vi "Clean Buffers.vi"(8 "error in (no error)":errorcluster, 11 "State In":T1) -> (0 "error out":errorcluster, 3 "State Out":T1)   [LabVIEW 2020, in "TDMS DAQ.lvlib" / "TDMS DAQ.lvclass"]
uses:
  TDMS DAQ.lvclass
  Helper Loop State.ctl
  <vilib>/Natan Biesmans/G2CPU GPU and CPU HPC Toolkit/G2CPU Libraries/Async IO/DMA Manager/DMA Manager.lvclass
  Configure TDMS DAQ.ctl
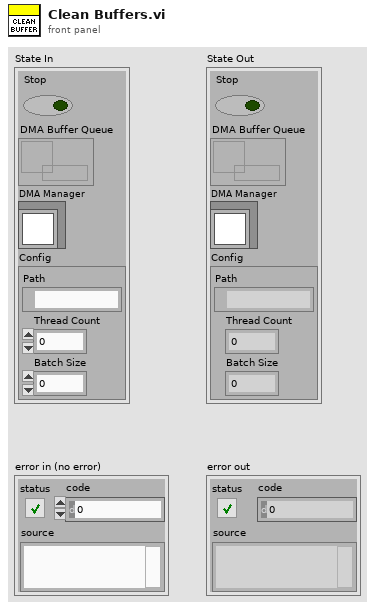
[diagram p1: front panel]
types:
  T1 = typedef "TDMS DAQ.lvlib/TDMS DAQ.lvclass/Helper Loop State.ctl" = cluster{"Stop":bool, "DMA Buffer Queue":refnum<queue>, "DMA Manager":refnum<class "DMA Manager.lvclass">, "Config":T2}
  T2 = typedef "TDMS DAQ.lvlib/TDMS DAQ.lvclass/Configure TDMS DAQ.ctl" = cluster{"Path":path, "Thread Count":i32, "Batch Size":i32}
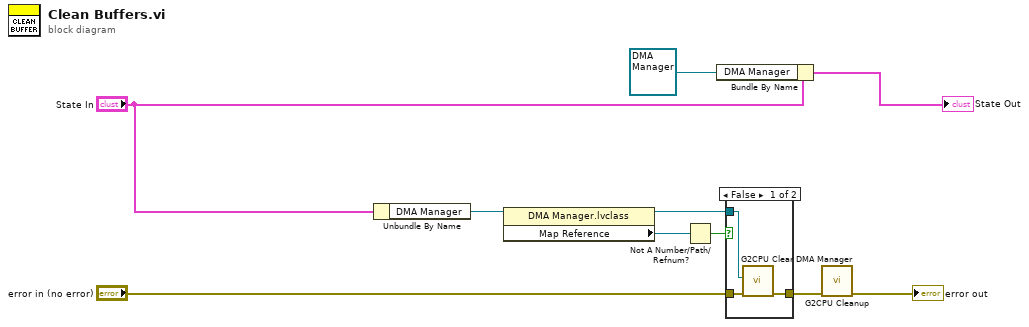
[diagram p0: block diagram]
diagram:
  n1 = Unbundle By Name("State In") -> ("DMA Manager"=w5:refnum<class "DMA Manager.lvclass">)
  n2 = property class="DMA Manager.lvclass"(reference=w5) -> (reference out=w1:refnum<class "DMA Manager.lvclass">, "Map Reference"=w3:refnum<data-value>)  [unwired: 1 in, 1 out]
  n3 = Not A Number/Path/Refnum?(number/path/refnum=w3) -> (NaN/Path/Refnum?=w2:bool)
  n4 = Bundle By Name(cluster="State In", "DMA Manager"=refnum<class "DMA Manager.lvclass"> refnum) -> (→"State Out":T1)
  n5 = case shown="False" w2 {
    tunnel: "error in (no error)" -> [w13 w14]
    tunnel: [w12 w14] -> w4
    tunnel: w1 -> [w11 _]
    frame False {
      n6 = call <vilib>:"G2CPU Clear DMA Manager.vi"("error in (no error)"=w13, "DMA Manager"=w11) -> ("error out"=w12:errorcluster)  [unwired: 9 in]
    }
    frame True {
    }
  }
  n7 = call <vilib>:"G2CPU Cleanup.vi"("error in (no error)"=w4) -> ("error out"=→"error out":errorcluster)  [unwired: 10 in]
